vi "libssh2_userauth_list.vi"(8 "error in (no error)":errorcluster, 10 "username":string, 11 "session":T1) -> (0 "error out":errorcluster, 2 "supported authentication schemes":string)   [LabVIEW 2013, in "libssh2.lvlib"]
doc: "Get a list of authentication methods that are available for a session.\n\nSends a SSH_USERAUTH_NONE request to the remote host. Unless the remote is configured to accept \"none\" as a viable authentication scheme, it will return SSH_USERAUTH_FAILURE along with a listing of what authentication schemes it does support. In the unlikely event that none-authentication succeeds, this method returns an empty string. This can be distinguished from a failing case by examining <B>libssh2_userauth_authenticated</B>."
uses:
  libssh2.lvlib
  Session Refnum.ctl
  Not A Session.vi
  <vilib>/Utility/error.llb/Error Cluster From Error Code.vi
  Global Settings.vi
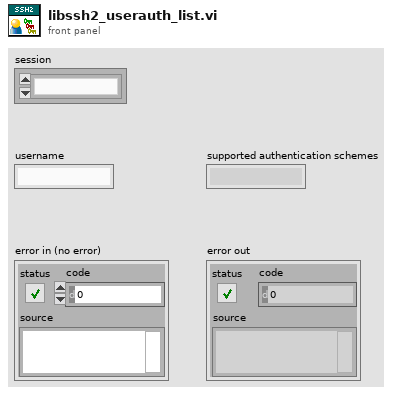
[diagram p1: front panel]
types:
  T1 = typedef "libssh2.lvlib/Session Refnum.ctl" = refnum<k1>
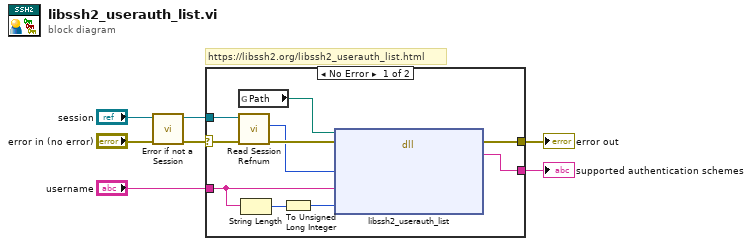
[diagram p0: block diagram]
diagram:
  # "https://libssh2.org/libssh2_userauth_list.html"
  n1 = call "Error if not a Session.vi"("error in (no error)"="error in (no error)", "session"="session") -> ("error out"=w3:errorcluster, "session out"=w1:T1)  [unwired: 8 in]
  n2 = case shown="No Error" w3 {
    selector: w3 -> [w14 w18]
    tunnel: "username" -> [w17 _]
    tunnel: [w16 _] -> w6
    tunnel: [w15 w18] -> w5
    tunnel: w1 -> [w13 _]
    frame No Error {
      n3 = global read "Global Settings.vi" "Path"() -> (w8:path)
      n4 = call "Read Session Refnum.vi"("error in (no error)"=w14, "session"=w13) -> ("error out"=w10:errorcluster, "LIBSSH2_SESSION*"=w9:u64)  [unwired: 5 in, 3 out]
      n5 = String Length(string=w17) -> (length=w11:i32)
      n6 = To Unsigned Long Integer(number=w11) -> (unsigned 32bit integer=w12:u32)
      n7 = dll-call lib="?" fn="libssh2_userauth_list"(path in=w8, error in=w10, "session"=w9, "username"=w17, "username_len"=w12) -> (error out=w15:errorcluster, "return value"=w16:string)  [unwired: 4 in, 1 out]
    }
    frame Error {
    }
  }
  "supported authentication schemes" <- w6
  "error out" <- w5
